vi "ESP_RT_UDP_init.vi"(0 "Trigger Port":tag, 1 "PXI(local) IP":string="192.168.1.188", 2 "ESP(remote) IP":string="192.168.1.182", 3 "error in":errorcluster) -> (7 "task out":refnum<k21>, 9 "connection ID out":refnum<k16>, 10 "error out":errorcluster)   [LabVIEW 2021]
uses:
  <vilib>/DAQmx/create/channels.llb/DAQmx Create Channel (DO-Digital Output).vi
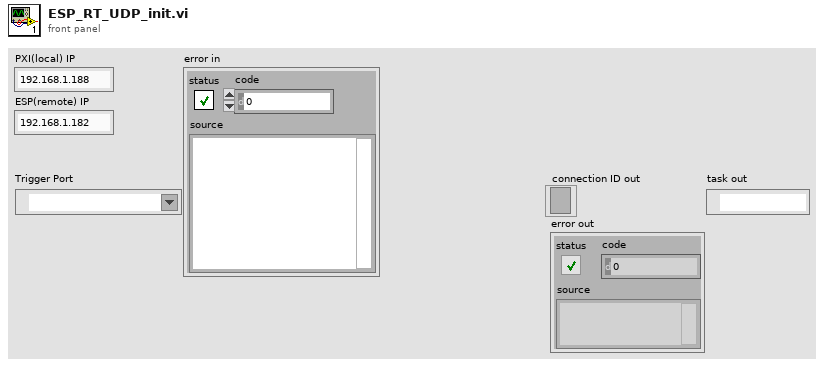
[diagram p1: front panel]
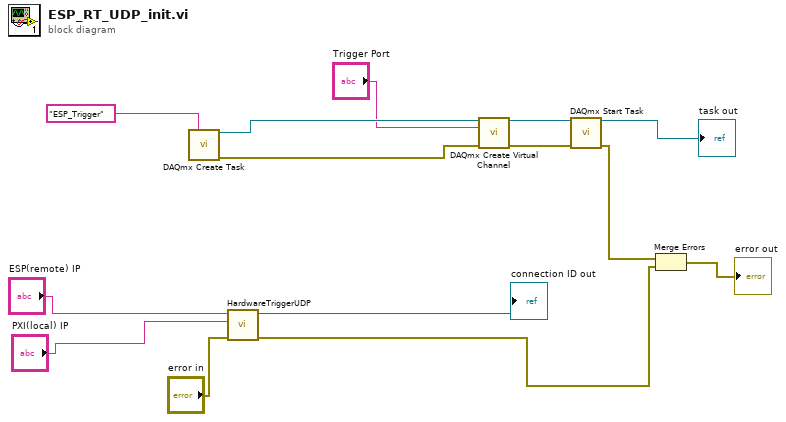
[diagram p0: block diagram]
diagram:
  n1 = call <vilib>:"DAQmx Create Task.vi"("new task name"="ESP_Trigger") -> ("task out"=w13:refnum<k21>, "error out"=w12:errorcluster)  [unwired: 13 in]
  n2 = call "HardwareTriggerUDP.vi"("error in"="error in", "Local IP address"="PXI(local) IP", "Remote IP address"="ESP(remote) IP") -> ("error out"=w8:errorcluster, "connection ID out"=→"connection ID out":refnum<k16>)  [unwired: 7 in]
  n3 = call-poly <vilib>:"DAQmx Create Virtual Channel.vi"("task in"=w13, "lines"="Trigger Port", "error in"=w12) -> ("task out"=w11:refnum<k21>, "error out"=w10:errorcluster)  [unwired: 11 in]
  n4 = call <vilib>:"DAQmx Start Task.vi"("task/channels in"=w11, "error in"=w10) -> ("task out"=→"task out":refnum<k21>, "error out"=w7:errorcluster)  [unwired: 12 in]
  n5 = Merge Errors(w7, w8) -> (→"error out":errorcluster)
